vi "Read PC Beamage.vi"(8 "error in":errorcluster) -> (0 "error out":errorcluster, 2 "Reply":string)   [LabVIEW 2009]
uses:
  BeamageNP.dll
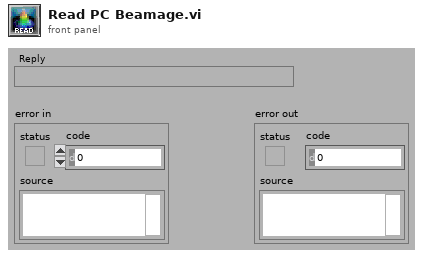
[diagram p1: front panel]
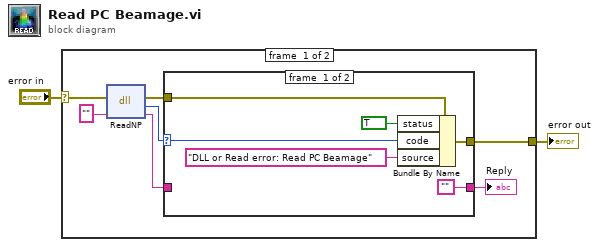
[diagram p0: block diagram]
diagram:
  n1 = case shown="No Error" "error in" {
    selector: "error in" -> [w8 w18]
    tunnel: [w5 w18] -> w1
    frame #0 {
      n2 = dll-call lib="S:/LabView Files/Beamage 3.0/BeamageNP.dll" fn="ReadNP"(error in=w8, "command"="") -> (error out=w6:errorcluster, "success"=w7:i32, "command"=w4:string)  [unwired: 2 in, 1 out]
      n3 = case shown="0, Default" w7 {
        selector: w7 -> [w11 _]
        tunnel: w6 -> [w14 w17]
        tunnel: [w13 w17] -> w5
        tunnel: w4 -> [_ w16]
        tunnel: ["" w16] -> w3
        frame #0 {
          n4 = Bundle By Name(cluster=w14, "status"=TRUE, "code"=w11, "source"="DLL or Read error: Read PC Beamage") -> (w13:errorcluster)
        }
        frame #1 {
          # "No error"
        }
      }
      "Reply" <- w3
    }
    frame #1 {
    }
  }
  "error out" <- w1
